vi "svx_Polar_Plot_CursorInfoVis_Read.vi"(4 "error in (no error)":errorcluster, 6 "Container State":T2, 7 "Display State In":T1) -> (0 "error out":errorcluster, 2 "Value":bool, 3 "Display State Out":T1)   [LabVIEW 2017, in "SVX Polar Plot.xctl"]
uses:
  <vilib>/addons/_XControls/Polar Plot/SVX Polar Plot.xctl
  <vilib>/_xctls/Container State.ctl
  <vilib>/addons/_XControls/Polar Plot/subVIs/svx_Polar_Plot_State.ctl
  <vilib>/addons/_XControls/Polar Plot/subVIs/svx_Polar_Plot_Internal_State.ctl
  <vilib>/addons/_XControls/Polar Plot/subVIs/svx_Polar_Indication_Arcs.ctl
  <vilib>/addons/_XControls/Polar Plot/subVIs/svx_Polar_Customized_Markers.ctl
  <vilib>/_xctls/XControlSupport.lvlib
panel:
  # "Replace the Value Indicator below with an Indicator of desired type.\nDo not remove this Indicator or the others from the connector pane. \nDo not change the connector pane pattern.\nThe Value Indicator should always be the second terminal from top on the output side in the connector pane."
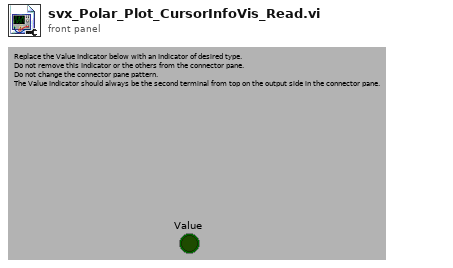
[diagram p1: front panel]
types:
  T1 = typedef "SVX Polar Plot.xctl/svx_Polar_Plot_State.ctl" = cluster{"Current State":refnum<queue>, "Previous State":variant}
  T2 = typedef "XControlSupport.lvlib/Container State.ctl" = cluster{"Indicator?":bool, "Run Mode?":bool, " Refnum":refnum<vi>}
  T3 = typedef "SVX Polar Plot.xctl/svx_Polar_Plot_Internal_State.ctl" = cluster{"Property Name":string[], "Container bounds":cluster{"Width":u32, "Height":u32}, "Scale range":cluster{"Maximum":dbl, "Increment":dbl}, "PointIdx":i32, "Marker list":cluster{"Name":string, "Color":u32, "Style":u8, "Point Style":u8, "Name Visible":bool, "Allow Drag":bool, "Annotation Mode":u32, "Plot":i32, "Index":i32, "Position":cluster{"X":dbl, "Y":dbl}, "X Scale":u32, "Y Scale":u32, "Show Arrow":bool, "Lock Name":bool, "Plot Area":i32, "Label Offset":cluster{"X":dbl, "Y":dbl}}[], "Color settings":cluster{"Arrow color":u32, "Magnitude major grid":u32, "Magnitude minor grid":u32, "Phase grid":u32, "Phase scale marker text":u32}, "Magnitude scale name":string, "Magnitude scale format string":string, "MagnitudeScale:Visible":bool, "MagnitudeScaleLabel:Visible":bool, "PhaseScale:Visible":bool, "Marker:Visible":bool, "Cursor:Visible":bool, "CursorName:Visible":bool, "Autoscale":bool, "Marker color":u32, "Line color":u32, "Cursor color":u32, "Magnitude scale marker color":u32, "Plot.Line Style":i32, "Plot.Line Width":i32, "Plot.Point Style":i32, "Cursor.Line Style":i32, "Cursor.Line Width":i32, "Cursor.Point Style":i32, "Cursor.Style":i32, "Marker.Point Style":i32, "Point/fill color":u32, "Background color":u32, "Cursor name":string, "Cursor Release":refnum<user-event>, "Scale Range Change":refnum<user-event>, "data size(s)":i32[], "Selectors:Visible":bool, "Selector:ring Strings":cluster{"Selector:Custom Strings":bool, "Selector:Row Strings []":string[], "Selector:Column Strings []":string[], "User:Row Strings []":string[], "User:Column Strings []":string[]}, "Lock Cursor Info Position":bool, "CursLoc":cluster{"magnitude":dbl, "phase":dbl, "time/rev/RPM":dbl}, "Plot Area:Position":cluster{"Left":i32, "Top":i32}, "Plot Area:Size":cluster{"Width":u32, "Height":u32}, "Marker.Style":i32, "Indication Arcs":T4, "Arc.Selector":u16, "customized marker":T5, "tree Width":u32, " Parents Tags":string[], "Children Tags":string[], "open?":bool[], "index":cluster{"row index":i32, "column index":i32}[], "Label":string, "custom strings changed":bool, "Owning VI":refnum<vi>, "Legend BG color":u32, "Legend font color":u32, "column Width":u32, "attribute":variant}
  T4 = typedef "SVX Polar Plot.xctl/svx_Polar_Indication_Arcs.ctl" = cluster{"Name":string, "Start radius":dbl, "End radius":dbl, "Line Style":i32, "Line Width":i32, "Border color":u32, "Fill color":u32, "Start angle":i16, "End angle":i16, "Visible":bool}[]
  T5 = typedef "SVX Polar Plot.xctl/svx_Polar_Customized_Markers.ctl" = cluster{"Name":string, "Color":u32, "Style":u8, "Point Style":u8, "Name Visible":bool, "Allow Drag":bool, "Annotation Mode":u32, "Plot":i32, "Index":i32, "Position":cluster{"Magnitude":dbl, "Phase":dbl}, "X Scale":u32, "Y Scale":u32, "Show Arrow":bool, "Lock Name":bool, "Plot Area":i32, "Label Offset":cluster{"Magnitude":dbl, "Phase":dbl}}[]
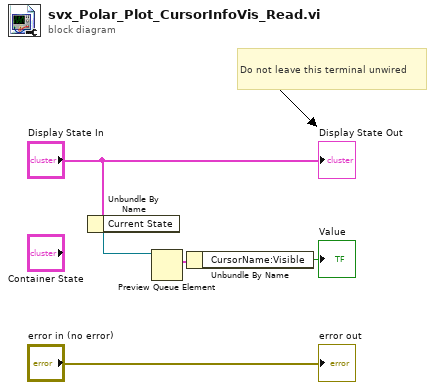
[diagram p0: block diagram]
diagram:
  # "Do not leave this terminal unwired"
  n1 = Unbundle By Name("Display State In") -> ("Current State"=w3:refnum<queue>)
  n2 = Preview Queue Element(queue=w3) -> (element=w2:T3)  [unwired: 2 in, 3 out]
  n3 = Unbundle By Name(w2) -> ("CursorName:Visible"=→"Value":bool)
  "error out" <- "error in (no error)"
  "Display State Out" <- "Display State In"
